vi "SaveVNAData.vi"(0 "Savingfolder":path caption="Saving folder", 1 "ScanStep":i32[](array[numeric]), 2 "VNA Freq":dbl[](array[numeric]), 3 "VNA Data":dbl[][](array[numeric]), 4 "error in (no error)":errorcluster) -> (5 "error out":errorcluster)   [LabVIEW 2017]
uses:
  <vilib>/Utility/file.llb/Write Delimited Spreadsheet (DBL).vi
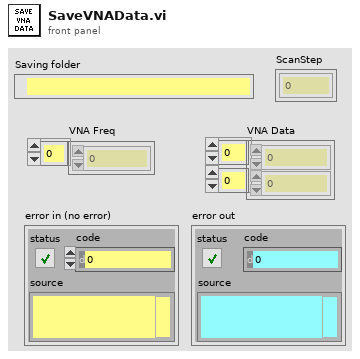
[diagram p1: front panel]
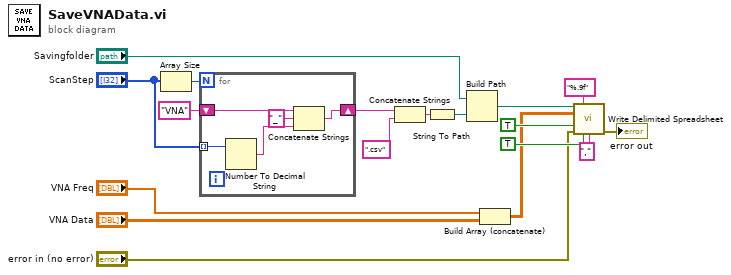
[diagram p0: block diagram]
diagram:
  n1 = Array Size(array="ScanStep") -> (size(s)=w11:i32)
  n2 = for {
    N: w11 -> [_]
    shift-right: [w20] -> w9
    shift-left: "VNA" ("string") -> [w21]
    tunnel: "ScanStep" -> [w19] mode=indexing
    n3 = Number To Decimal String(number=w19) -> (decimal integer string=w22:string)  [unwired: 1 in]
    n4 = Concatenate Strings(w21, "_", w22) -> (w20:string)
  }
  n5 = Concatenate Strings(w9, ".csv") -> (w14:string)
  n6 = String To Path(string=w14) -> (path=w13:path)
  n7 = Build Path(base path="Savingfolder", name or relative path=w13) -> (appended path=w16:path)
  n8 = Build Array (concatenate)("VNA Freq", "VNA Data") -> (w7:dbl[][])
  n9 = call-poly <vilib>:"Write Delimited Spreadsheet.vi"("file path (dialog if empty)"=w16, "format (%.3f)"="%.9f", "2D data"=w7, "append to file? (new file:F)"=TRUE, "error in (no error)"="error in (no error)", "transpose? (no:F)"=TRUE ("transpose? (F)"), "delimiter (\\t)"="," ("delimiter (\\t)")) -> ("error out"=→"error out":errorcluster)  [unwired: 7 in, 1 out]
